vi "ProcessState-Stopped.vi"(3 "ProcessStateNotifier in":refnum<notifier>, 9 "error in (no error)":errorcluster) -> (6 "error out":errorcluster)   [LabVIEW 2009]
uses:
  ProcessState.ctl
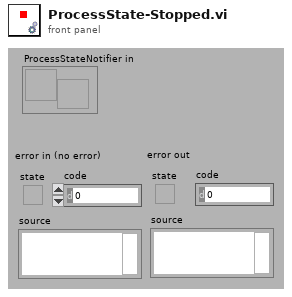
[diagram p1: front panel]
types:
  T1 = typedef "ProcessState.ctl" = enum16{"STARTING", "RUNNING", "STOPPING", "STOPPPED"}
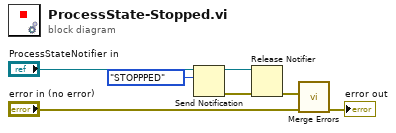
[diagram p0: block diagram]
diagram:
  n1 = Send Notification(notification=ProcessState."STOPPPED", notifier="ProcessStateNotifier in") -> (notifier out=w5:refnum<notifier>, error out=w4:errorcluster)  [unwired: 1 in]
  n2 = Release Notifier(notifier=w5, error in (no error)=w4) -> (error out=w1:errorcluster)  [unwired: 3 out]
  n3 = call <vilib>:"Merge Errors.vi"("error in 3 (no error)"="error in (no error)", "error in 2 (no error)"=w1) -> ("error out"=→"error out":errorcluster)  [unwired: 2 in, 3 out]
